vi "GetParent.vi"(8 "error in (no error)":errorcluster, 10 "Tag":string, 11 "ResultTree in":refnum<class "ResultTree.lvclass">) -> (0 "error out":errorcluster, 2 "Parent Tag":string, 3 "ResultTree out":refnum<class "ResultTree.lvclass">)   [LabVIEW 2019, in "ResultTree.lvclass"]
doc: "Returns the parent tag for a given tag name."
uses:
  ResultTree.lvclass
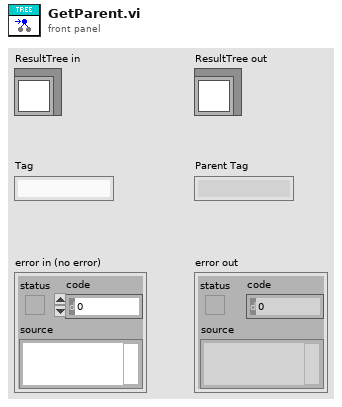
[diagram p1: front panel]
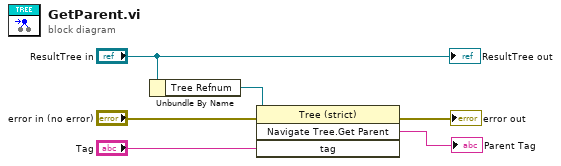
[diagram p0: block diagram]
diagram:
  n1 = Unbundle By Name("ResultTree in") -> ("Tree Refnum"=w5:refnum<vi>)
  n2 = invoke class="Tree (strict)" method="Navigate Tree.Get Parent"(reference=w5, error in="error in (no error)", "tag"="Tag") -> (error out=→"error out":errorcluster, "Navigate Tree:Get Parent"=→"Parent Tag":string)  [unwired: 1 in, 2 out]
  "ResultTree out" <- "ResultTree in"
